vi "Z_Alignment_v11 (SubVI).vi"(4 "System no.":i32, 5 "Z range":dbl, 6 "Intensity Graph":dbl[][](array[numeric]), 7 "Z Mesh":dbl, 8 "error in (no error)":errorcluster, 9 "Z":dbl, 10 "Y":dbl, 11 "X":dbl) -> (0 "error out":errorcluster)   [LabVIEW 2023]
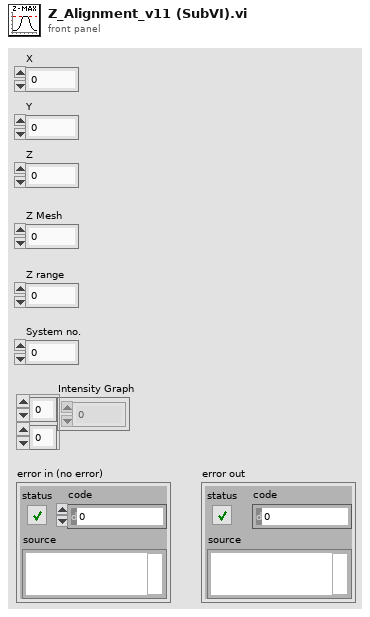
[diagram p1: front panel]
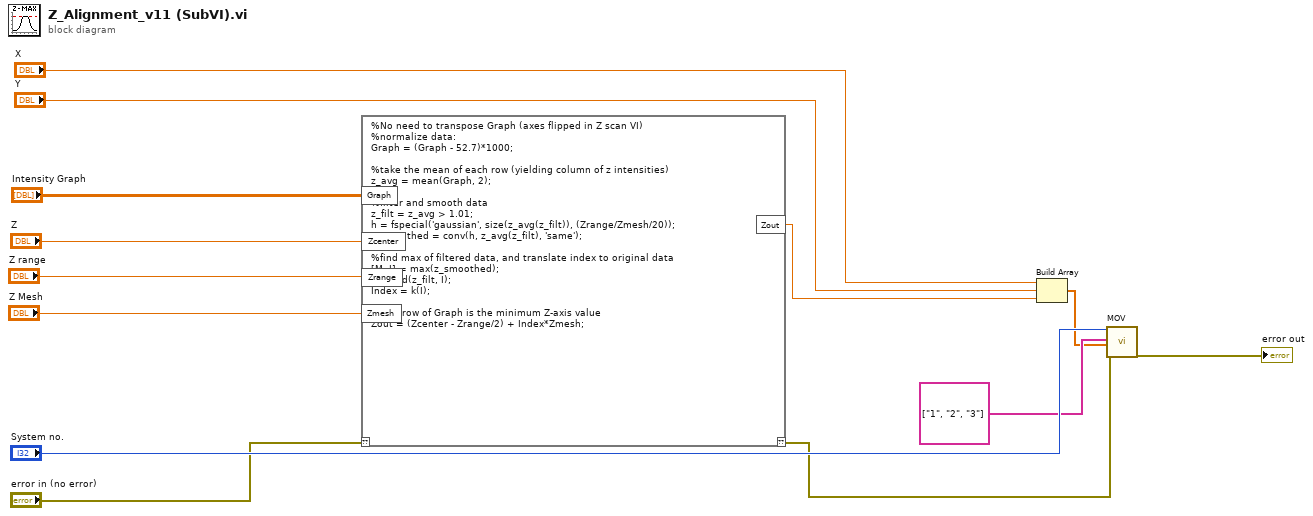
[diagram p0: block diagram]
diagram:
  n1 = script code="%No need to transpose Graph (axes flipped in Z scan VI)\n%normalize data:\nGraph = (Graph - 52.7)*1000;\n\n%take the mean of each row (yielding column of z intensities)\nz_avg = mean(Graph, 2);\n\n%filter and smooth data\nz_filt = z_avg > 1.01;\nh = fspecial('gaussian', size(z_avg(z_filt)), (Zrange/Zmesh/20));\nz_smoothed = conv(h, z_avg(z_filt), 'same');\n\n%find max of filtered data, and translate index to original data\n[M, I] = max(z_smoothed);\nk = find(z_filt, I);\nIndex = k(I);\n\n%first row of Graph is the minimum Z-axis value\nZout = (Zcenter - Zrange/2) + Index*Zmesh;"("??"="error in (no error)", "Graph"="Intensity Graph", "Zcenter"="Z", "Zrange"="Z range", "Zmesh"="Z Mesh") -> ("??"=w1:errorcluster, "Zout"=w3:dbl)
  n2 = Build Array("X", "Y", w3) -> (w8:dbl[])
  n3 = call "MOV.vi"("System no."="System no.", "Axes to move"=string[] ["1", "2", "3"], "Position values"=w8, "error in"=w1) -> ("error out"=→"error out":errorcluster)  [unwired: 1 in, 14 out]
